vi "Symphony Init ADC & Gain.vi"(8 "error in (no error)":errorcluster, 11 "JYCCDLib.IJYCCDReqd":refnum<k7>) -> (0 "error out":errorcluster, 1 "ADC Values":T1(array[cluster]), 2 "Gain Values":T1(array[cluster]), 3 "JYCCDLib.IJYCCDReqd Out":refnum<k7>, 4 "CurrentADC":i32, 5 "CurrentGain":i32)   [LabVIEW 2012]
panel:
  out "Gain description":string[](array[string])
  out "Gain Number":i32[](array[numeric])
  out "ADC description":string[](array[string])
  out "ADC Number":i32[](array[numeric])
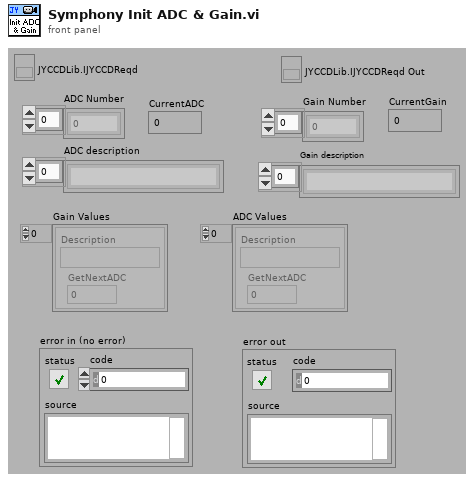
[diagram p1: front panel]
types:
  T1 = cluster{"Description":string, "GetNextADC":u16}[]
  T2 = enum16{"GetFirstADC", "GetNextADC", "GetFirstGain", "GetNextGain", "Init Done", "Error"}
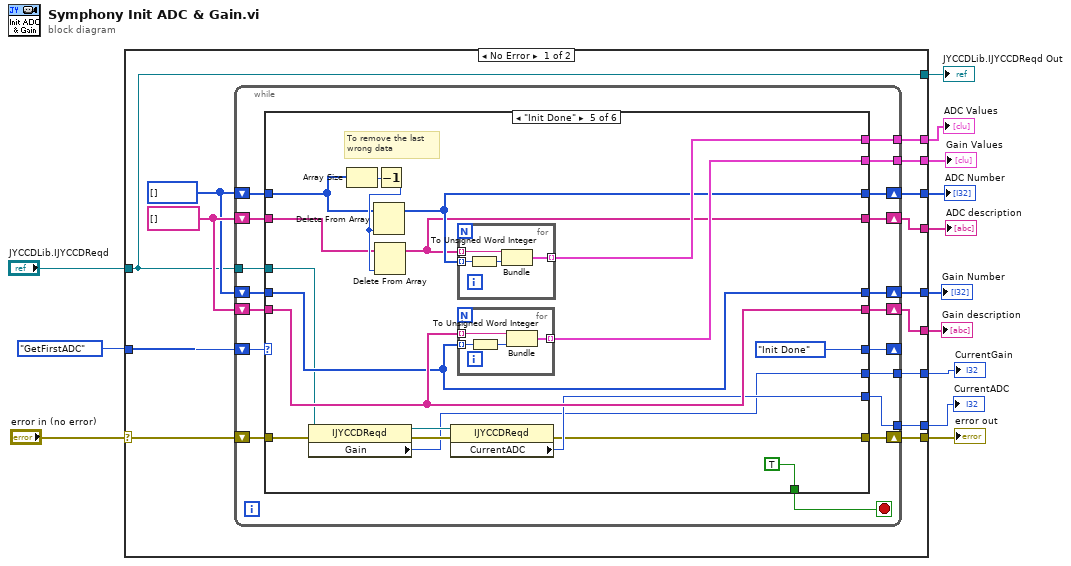
[diagram p0: block diagram]
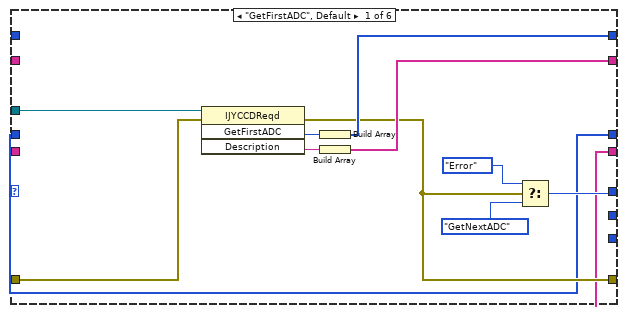
[diagram p2: hidden frame]
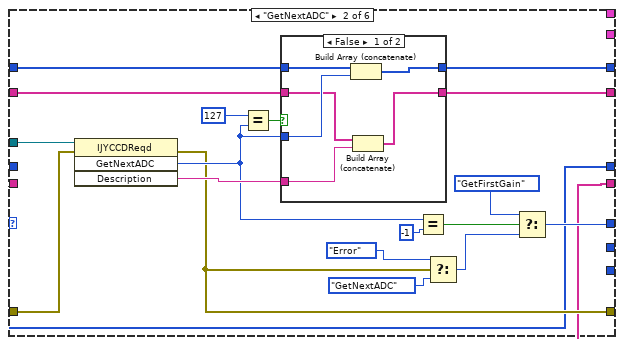
[diagram p3: hidden frame]
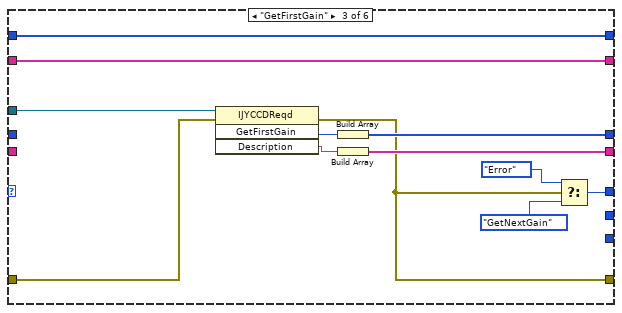
[diagram p5: hidden frame]
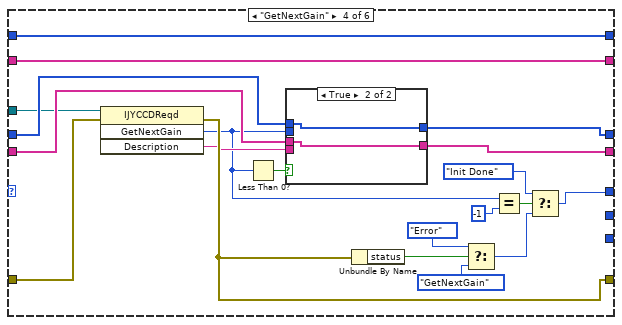
[diagram p6: hidden frame]
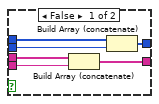
[diagram p7: hidden frame]
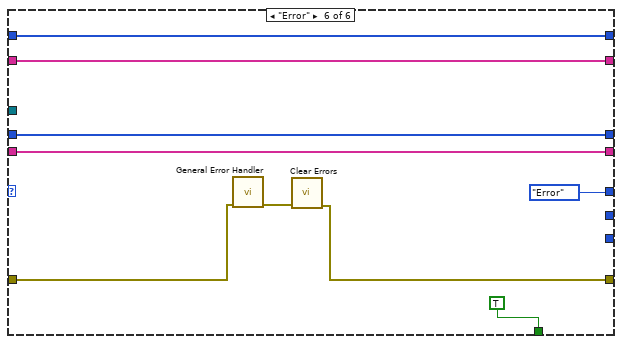
[diagram p8: hidden frame]
diagram:
  n1 = case shown="No Error" "error in (no error)" {
    selector: "error in (no error)" -> [w26 w163]
    tunnel: "JYCCDLib.IJYCCDReqd" -> [w14 w162]
    tunnel: T2."GetFirstADC" -> [w27 _]
    tunnel: [w25 w163] -> w11
    tunnel: [w22 _] -> w9
    tunnel: [w21 _] -> w8
    tunnel: [w14 w162] -> w7
    tunnel: [w20 _] -> w6
    tunnel: [w19 _] -> w5
    tunnel: [w18 _] -> w4
    tunnel: [w17 _] -> w3
    tunnel: [w16 _] -> w2
    tunnel: [w15 _] -> w1
    frame No Error {
      w23 = i32[] []
      w24 = string[] []
      n2 = while {
        shift-right: [w38] -> _
        shift-left: w27 -> [w45]
        shift-right: [w37] -> w25
        shift-left: w26 -> [w44]
        tunnel: w14 -> [w43]
        shift-right: [w42] -> w22
        shift-left: w23 -> [w40]
        shift-right: [w41] -> w21
        shift-left: w24 -> [w39]
        shift-right: [w35] -> w19
        shift-left: w24 -> [w33]
        shift-right: [w36] -> w20
        shift-left: w23 -> [w34]
        tunnel: [w31] -> w18
        tunnel: [w30] -> w17
        tunnel: [w29] -> w16
        tunnel: [w28] -> w15
        stop <- w32 stop-if-true
        n3 = case shown="\"Init Done\"" w45 {
          tunnel: w44 -> [w54 w73 w94 w112 w137 w160]
          tunnel: w43 -> [w55 w74 w95 w113 w138 _]
          tunnel: [w53 w67 w86 w115 w131 w156] -> w42
          tunnel: [w52 w68 w87 w101 w129 w155] -> w41
          tunnel: w40 -> [_ w72 w86 w115 w132 w156]
          tunnel: w39 -> [_ w71 w87 w101 w130 w155]
          tunnel: [w51 w64 w88 w102 T2."Init Done" T2."Error"] -> w38
          tunnel: [w50 w63 w89 w103 w126 w158] -> w37
          tunnel: [w47 w59 w93 w111 w139 w154] -> w36
          tunnel: [w46 w58 w92 w110 w140 w153] -> w35
          tunnel: w34 -> [w47 w59 _ w116 w139 w154]
          tunnel: w33 -> [w46 w58 _ w114 w140 w153]
          tunnel: [_ _ _ _ TRUE TRUE] -> w32
          tunnel: [_ _ _ _ w142 _] -> w31
          tunnel: [_ _ _ _ w141 _] -> w30
          tunnel: [_ _ _ _ w127 _] -> w29
          tunnel: [_ _ _ _ w128 _] -> w28
          frame "GetFirstADC", Default {
            n4 = invoke class="IJYCCDReqd" method="GetFirstADC"(reference=w55, error in=w54) -> (error out=w50:errorcluster, "GetFirstADC"=w57:i32, "Description"=w56:string)  [unwired: 2 in, 1 out]
            n5 = Build Array(w57) -> (w53:i32[])
            n6 = Build Array(w56) -> (w52:string[])
            n7 = Select(t=T2."Error", s=w50, f=T2."GetNextADC") -> (s? t:f=w51:T2)
          }
          frame "GetNextADC" {
            n8 = invoke class="IJYCCDReqd" method="GetNextADC"(reference=w74, error in=w73) -> (error out=w63:errorcluster, "GetNextADC"=w70:i32, "Description"=w77:string)  [unwired: 2 in, 1 out]
            n9 = Equal?(x=127 ("y"), y=w70) -> (x = y?=w76:bool)
            n10 = case shown="False" w76 {
              tunnel: w72 -> [w83 w84]
              tunnel: w70 -> [w82 _]
              tunnel: w71 -> [w81 w85]
              tunnel: w77 -> [w80 _]
              tunnel: [w79 w84] -> w67
              tunnel: [w78 w85] -> w68
              frame False {
                n11 = Build Array (concatenate)(w83, w82) -> (w79:i32[])
                n12 = Build Array (concatenate)(w81, w80) -> (w78:string[])
              }
              frame True {
              }
            }
            n13 = Equal?(x=w70, y=-1) -> (x = y?=w65:bool)
            n14 = Select(t=T2."Error", s=w63, f=T2."GetNextADC") -> (s? t:f=w66:T2)
            n15 = Select(t=T2."GetFirstGain", s=w65, f=w66) -> (s? t:f=w64:T2)
          }
          frame "GetFirstGain" {
            n16 = invoke class="IJYCCDReqd" method="GetFirstGain"(reference=w95, error in=w94) -> (error out=w89:errorcluster, "GetFirstGain"=w96:i32, "Description"=w97:string)  [unwired: 2 in, 1 out]
            n17 = Build Array(w96) -> (w93:i32[])
            n18 = Build Array(w97) -> (w92:string[])
            n19 = Select(t=T2."Error", s=w89, f=T2."GetNextGain") -> (s? t:f=w88:T2)
          }
          frame "GetNextGain" {
            n20 = invoke class="IJYCCDReqd" method="GetNextGain"(reference=w113, error in=w112) -> (error out=w103:errorcluster, "GetNextGain"=w98:i32, "Description"=w100:string)  [unwired: 2 in, 1 out]
            n21 = Less Than 0?(x=w98) -> (x < 0?=w99:bool)
            n22 = case shown="True" w99 {
              tunnel: w116 -> [w123 w125]
              tunnel: w114 -> [w122 w124]
              tunnel: [w121 w125] -> w111
              tunnel: [w120 w124] -> w110
              tunnel: w98 -> [w119 _]
              tunnel: w100 -> [w118 _]
              frame False {
                n23 = Build Array (concatenate)(w122, w118) -> (w120:string[])
                n24 = Build Array (concatenate)(w123, w119) -> (w121:i32[])
              }
              frame True {
              }
            }
            n25 = Unbundle By Name(w103) -> ("status"=w106:bool)
            n26 = Select(t=T2."Error", s=w106, f=T2."GetNextGain") -> (s? t:f=w104:T2)
            n27 = Equal?(x=w98, y=-1) -> (x = y?=w109:bool)
            n28 = Select(t=T2."Init Done", s=w109, f=w104) -> (s? t:f=w102:T2)
          }
          frame "Init Done" {
            # "To remove the last \nwrong data"
            n29 = property class="IJYCCDReqd"(reference=w138, error in=w137) -> (reference out=w135:refnum<k7>, error out=w136:errorcluster, "Gain"=w127:i32)
            n30 = Array Size(array=w132) -> (size(s)=w134:i32)
            n31 = Decrement(x=w134) -> (x-1=w133:i32)
            n32 = Delete From Array(array=w132, index=w133) -> (array with subset deleted=w131:i32[])  [unwired: 1 in, 1 out]
            n33 = Delete From Array(array=w130, index=w133) -> (array with subset deleted=w129:string[])  [unwired: 1 in, 1 out]
            n34 = property class="IJYCCDReqd"(reference=w135, error in=w136) -> (error out=w126:errorcluster, "CurrentADC"=w128:i32)  [unwired: 1 out]
            n35 = for {
              tunnel: w131 -> [w150] mode=indexing
              tunnel: w129 -> [w151] mode=indexing
              tunnel: [w152] -> w141 mode=indexing
              n36 = To Unsigned Word Integer(number=w150) -> (unsigned 16bit integer=w149:u16)
              n37 = Bundle("Description"=w151, w149) -> (w152:cluster{"Description":string, u16})  [unwired: 1 in]
            }
            n38 = for {
              tunnel: w139 -> [w146] mode=indexing
              tunnel: w140 -> [w147] mode=indexing
              tunnel: [w148] -> w142 mode=indexing
              n39 = To Unsigned Word Integer(number=w146) -> (unsigned 16bit integer=w145:u16)
              n40 = Bundle("Description"=w147, w145) -> (w148:cluster{"Description":string, u16})  [unwired: 1 in]
            }
          }
          frame "Error" {
            n41 = call <vilib>:"General Error Handler.vi"("error in (no error)"=w160) -> ("error out"=w159:errorcluster)  [unwired: 10 in, 4 out]
            n42 = call <vilib>:"Clear Errors.vi"("error in (no error)"=w159) -> ("error out"=w158:errorcluster)  [unwired: 6 in]
          }
        }
      }
    }
    frame Error {
    }
  }
  "JYCCDLib.IJYCCDReqd Out" <- w7
  "error out" <- w11
  "ADC Number" <- w9
  "ADC description" <- w8
  "Gain Number" <- w6
  "Gain description" <- w5
  "ADC Values" <- w3
  "Gain Values" <- w4
  "CurrentADC" <- w1
  "CurrentGain" <- w2
